vi "RS232Command.vi"(1 "OutputFIFO":refnum<k21>="DisplacementTxFIFO") -> ()   [LabVIEW 2016]
uses:
  <vilib>/rvi/interface/RandomDataEmulation/niFpgaRandomDataHandleErrors.vi
  <vilib>/rvi/DataTransferAndStorage/Container/Common/niFpgaContainerExecOnDevCompGetState.vi
  <vilib>/rvi/Emulation/niFpgaEmulationIsFPGAContextNoSignature.vi
  <vilib>/rvi/Emulation/niFpgaSctlEmulationGetInTimedLoop.vi
  <vilib>/rvi/errors/niFpgaSetErrorForExecOnDevCompSimple.vi
  <vilib>/rvi/eio/common/nirviEmuReportErrorAndStop.vi
  <vilib>/rvi/DataTransferAndStorage/Container/Common/niFpgaContainerGetUniqueNameForEmu.vi
  <vilib>/rvi/FIFO/Fifo_Resource/nirvififoEmulationSetSize.vi
  <vilib>/rvi/FIFO/Fifo_Resource/nirviFifoEmulationQueueMgr.vi
  <instcachedir>/0/nirviFifoEmulationQueueMgr_E5CAEC123FF24DC58D834DCA3CDAA9B5.lvgen/nirviFifoEmulationQueueMgr_E5CAEC123FF24DC58D834DCA3CDAA9B5_002.vi
  <vilib>/rvi/FIFO/Fifo_Resource/nirvififoEmulationDetermineInputValidOut.vi
  <vilib>/rvi/FIFO/Fifo_Resource/nirvififoEmulationCreateLock.vi
  <vilib>/rvi/Emulation/niFpgaProcessEmulError.vi
  <vilib>/rvi/FIFO/Fifo_Resource/nirvififoEmulationObtainLock.vi
  <vilib>/rvi/FIFO/Fifo_Resource/nirvififoEmulationReleaseLock.vi
  <vilib>/rvi/occurrence/nirviWaitOnOccurrenceBase.vi
  <vilib>/rvi/errors/nirviReportUnexpectedCaseInternalError.vi
  <vilib>/rvi/errors/nirviReportUnexpectedCaseInternalError (U32).vi
  <vilib>/Utility/error.llb/Clear Errors.vi
  <instcachedir>/0/nirviFifoEmulationQueueMgr_E5CAEC123FF24DC58D834DCA3CDAA9B5.lvgen/nirviFifoEmulationQueueMgr_E5CAEC123FF24DC58D834DCA3CDAA9B5_009.vi
  <vilib>/rvi/DataTransferAndStorage/Container/XNode/niFpgaContainer.xnode
  <vilib>/rvi/interface/RandomDataEmulation/nirviRandomDataFpgaReadWriteTemplate.vi
  <vilib>/rvi/FIFO/Fifo_Resource/niFpgaFifoEmulationRefIn.vi
  Common_FPGA_FIFO/FPGAFIFO.lvlib
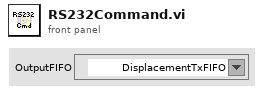
[diagram p1: front panel]
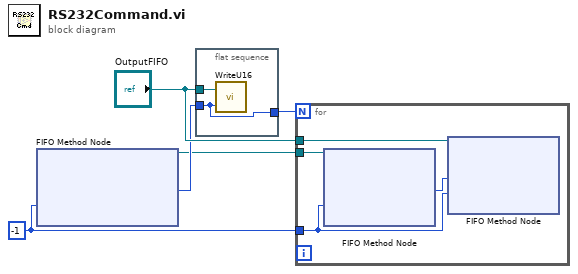
[diagram p0: block diagram]
diagram:
  w1 = -1 ("Timeout")
  n1 = xnode ("FIFO Method Node")("Timeout"=w1) -> ("Element"=w3:u16, "FIFO Out"=w2:refnum<k21>)  [unwired: 1 in, 1 out]
  n2 = flat-sequence {
    tunnel: w3 -> [w7]
    tunnel: [w7] -> w5
    tunnel: "OutputFIFO" -> [w6]
    frame #0 {
      n3 = call "WriteU16.vi"("U16"=w7, "FIFO"=w6) -> ()  [unwired: 1 in]
    }
  }
  n4 = for {
    N: w5 -> [_]
    tunnel: "OutputFIFO" -> [w10]
    tunnel: w2 -> [w9]
    tunnel: w1 -> [w8]
    n5 = xnode ("FIFO Method Node")("Timeout"=w8, "FIFO In"=w9) -> ("Element"=w11:u16)  [unwired: 2 out]
    n6 = xnode ("FIFO Method Node")("Element"=w11, "Timeout"=w8, "FIFO In"=w10) -> ()  [unwired: 2 out]
  }
